vi "2D-ShapeBuilder-INO.vi"(11 "Number of Sides":i32=3) -> (2 "Y out":dbl[](array[numeric])=[1.0, -0.4999999999999998, -0.5000000000000004, 1.0], 3 "X out":dbl[](array[numeric])=[0.0, 0.8660254037844387, -0.8660254037844384, 0.0])   [LabVIEW 2014]
doc: "André Romero - 2018\nandretec@ifsc.usp.br\n\n2D Shape Builder"
panel:
  out "Frequency (KHz)":ext
  out "interval time (us)":ext
  out "Delta Y":dbl[](array[numeric])=[-2999.9999999999995, -1.3642420526593924e-12, 3000.000000000001]
  out "Delta X":dbl[](array[numeric])=[1732.0508075688774, -3464.1016151377544, 1732.0508075688767]
  out "array w/ subset deleted 2":dbl[](array[numeric])=[-999.9999999999995, -1000.0000000000009, 2000.0]
  out "array w/ subset deleted":ext[](array[numeric])=[1732.0508075688774, -1732.0508075688767, 0.0]
  out "Vy":ext[](array[numeric])=[0.04330127018922192983, 1.9691137908567695728e-17, 0.04330127018922193538]
  out "Vx":ext[](array[numeric])=[0.025000000000000005552, 0.05, 0.024999999999999986123]
  in  "Velocidade (mm/s)":ext=0.05
  in  "Radius (steps)":dbl=2000.0
  out "XY Graph 2":cluster{dbl[], dbl[]}(graph)={[0.0, 1732.0508075688774, -1732.0508075688767, 0.0], [2000.0, -999.9999999999995, -1000.0000000000009, 2000.0]}
  out "Y":dbl[](array[numeric])=[2000.0, -999.9999999999995, -1000.0000000000009, 2000.0]
  out "X":dbl[](array[numeric])=[0.0, 1732.0508075688774, -1732.0508075688767, 0.0]
  out "XY Graph":cluster{dbl[], dbl[]}(graph)={[0.0, 0.8660254037844387, -0.8660254037844384, 0.0], [1.0, -0.4999999999999998, -0.5000000000000004, 1.0]}
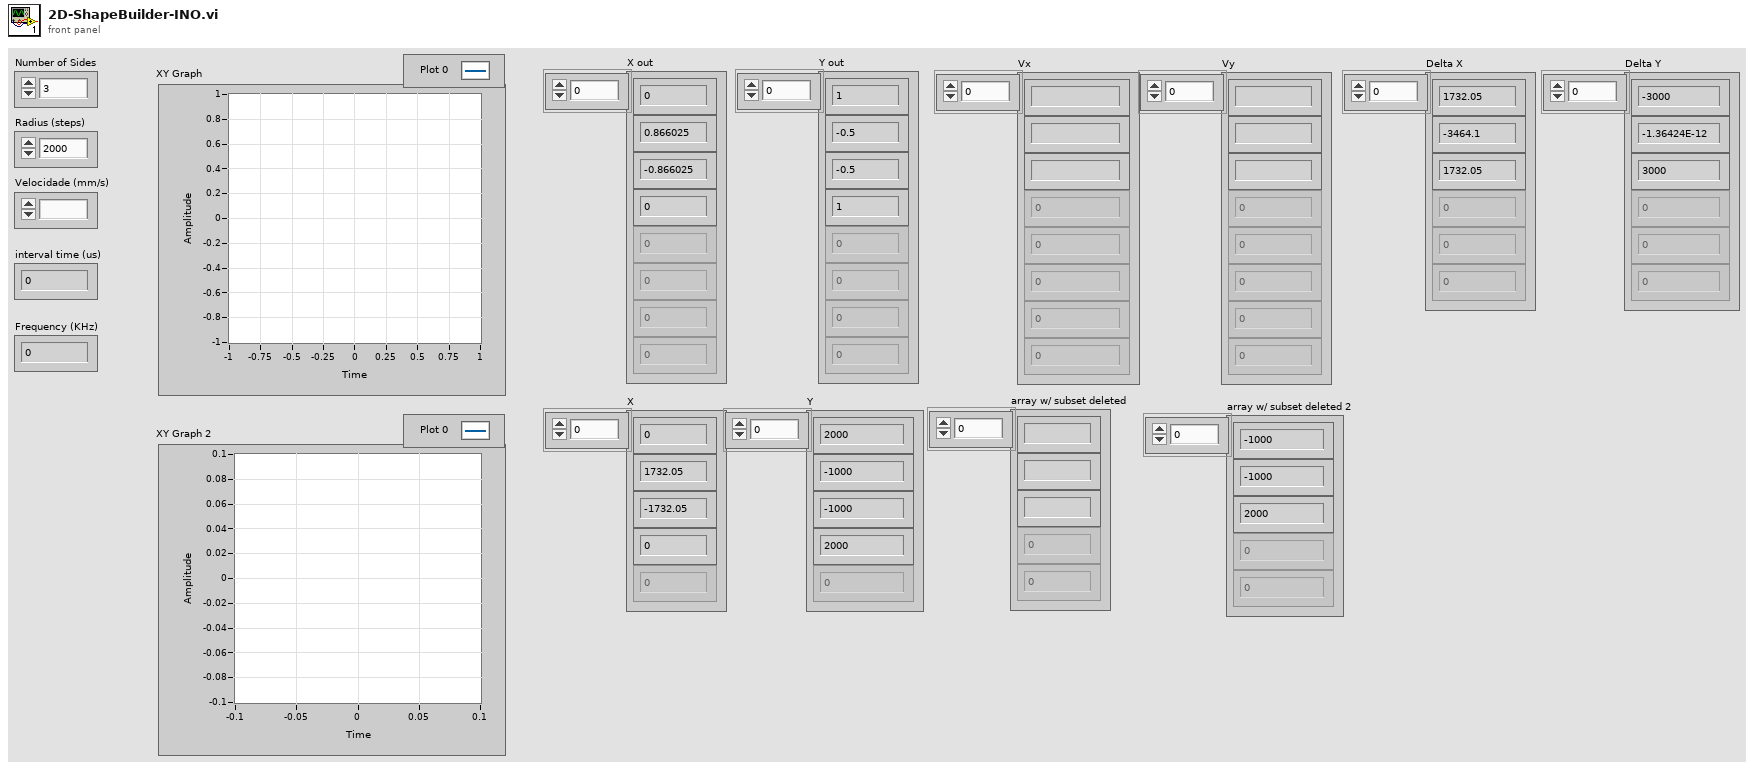
[diagram p1: front panel]
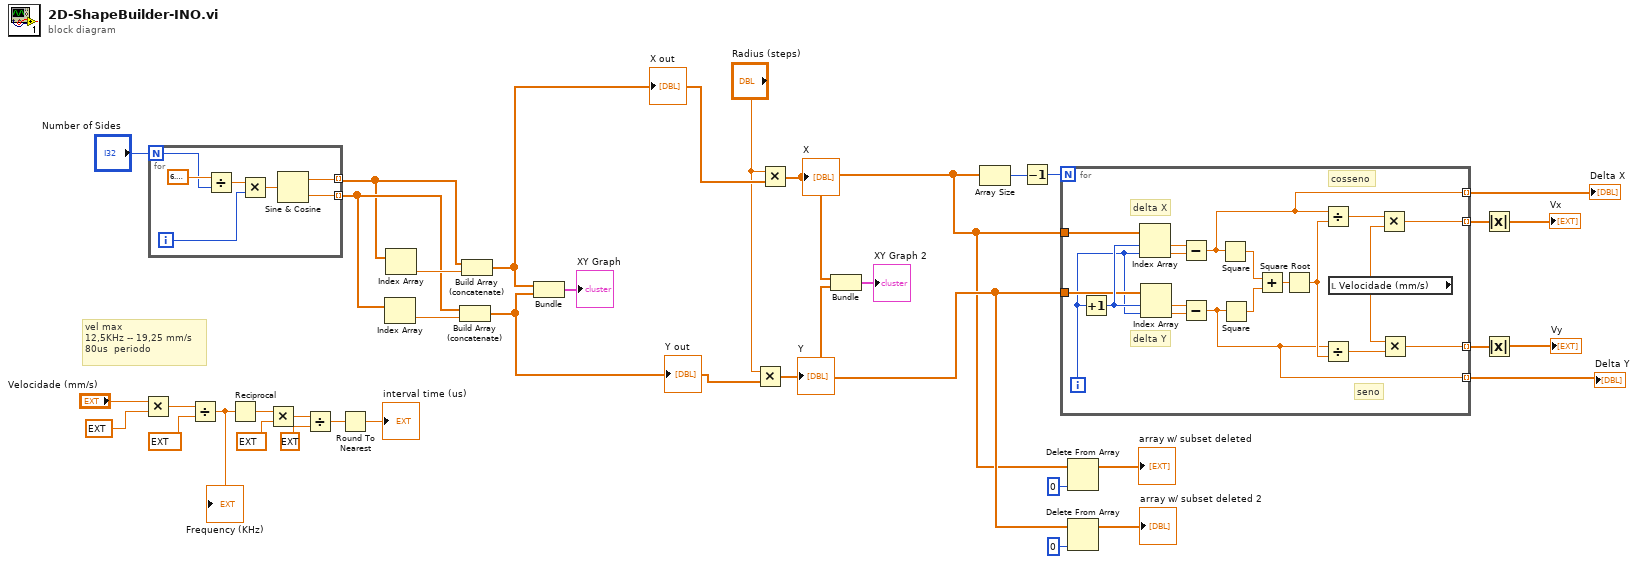
[diagram p0: block diagram]
diagram:
  # "vel max\n12,5KHz -- 19,25 mm/s\n80us  periodo"
  n1 = Multiply(x="Velocidade (mm/s)", y=ext 12.5) -> (x*y=w14:ext)
  n2 = for {
    N: "Number of Sides" -> [w41]
    tunnel: [w37] -> w30 mode=indexing
    tunnel: [w36] -> w31 mode=indexing
    i -> [w39]
    n3 = Divide(x=6.283185307179586, y=w41) -> (x/y=w40:dbl)
    n4 = Multiply(x=w40, y=w39) -> (x*y=w38:dbl)
    n5 = Sine & Cosine(0:w38) -> (1:w37:dbl, 2:w36:dbl)
  }
  n6 = Divide(x=w14, y=ext 19.25) -> (x/y=w12:ext)
  "Frequency (KHz)" <- w12
  n7 = Reciprocal(x=w12) -> (1/x=w11:ext)
  n8 = Multiply(x=w11, y=ext 1000.0) -> (x*y=w9:ext)
  n9 = Divide(x=w9, y=ext 2.0) -> (x/y=w7:ext)
  n10 = Round To Nearest(number=w7) -> (nearest integer value=→"interval time (us)":ext)
  n11 = Index Array(array=w31) -> (element=w32:dbl)  [unwired: 1 in]
  n12 = Index Array(array=w30) -> (element=w33:dbl)  [unwired: 1 in]
  n13 = Build Array (concatenate)(w31, w32) -> (w28:dbl[])
  "Y out" <- w28
  n14 = Build Array (concatenate)(w30, w33) -> (w29:dbl[])
  "X out" <- w29
  n15 = Bundle(w29, w28) -> (→"XY Graph":cluster{dbl[], dbl[]})  [unwired: 1 in]
  n16 = Multiply(x="Radius (steps)", y=w28) -> (x*y=w17:dbl[])
  "Y" <- w17
  n17 = Multiply(x="Radius (steps)", y=w29) -> (x*y=w5:dbl[])
  "X" <- w5
  n18 = Bundle(w5, w17) -> (→"XY Graph 2":cluster{dbl[], dbl[]})  [unwired: 1 in]
  n19 = Array Size(array=w5) -> (size(s)=w25:i32)
  n20 = Decrement(x=w25) -> (x-1=w22:i32)
  n21 = for {
    N: w22 -> [_]
    tunnel: w5 -> [w50]
    tunnel: w17 -> [w49]
    tunnel: [w47] -> w24 mode=indexing
    tunnel: [w46] -> w23 mode=indexing
    tunnel: [w45] -> w4 mode=indexing
    tunnel: [w44] -> w3 mode=indexing
    i -> [w48]
    # "seno"
    # "cosseno"
    # "delta Y"
    # "delta X"
    n22 = Increment(x=w48) -> (x+1=w61:i32)
    n23 = Index Array(array=w50, index #1=w61, index #2=w48) -> (element #1=w52:dbl, element #2=w59:dbl)
    n24 = Index Array(array=w49, index #1=w61, index #2=w48) -> (element #1=w51:dbl, element #2=w60:dbl)
    n25 = Subtract(x=w52, y=w59) -> (x-y=w45:dbl)
    n26 = Subtract(x=w51, y=w60) -> (x-y=w44:dbl)
    n27 = Square(x=w45) -> (x^2=w58:dbl)
    n28 = Square(x=w44) -> (x^2=w57:dbl)
    n29 = Add(x=w58, y=w57) -> (x+y=w56:dbl)
    n30 = Square Root(x=w56) -> (sqrt(x)=w55:dbl)
    n31 = Divide(x=w45, y=w55) -> (x/y=w54:dbl)
    n32 = Divide(x=w44, y=w55) -> (x/y=w53:dbl)
    n33 = local read "Velocidade (mm/s)"() -> (w43:ext)
    n34 = Multiply(x=w54, y=w43) -> (x*y=w47:ext)
    n35 = Multiply(x=w43, y=w53) -> (x*y=w46:ext)
  }
  "Delta X" <- w4
  "Delta Y" <- w3
  n36 = Delete From Array(array=w5, index=0) -> (array with subset deleted=→"array w/ subset deleted":dbl[])  [unwired: 1 in, 1 out]
  n37 = Delete From Array(array=w17, index=0) -> (array with subset deleted=→"array w/ subset deleted 2":dbl[])  [unwired: 1 in, 1 out]
  n38 = Absolute Value(x=w24) -> (abs(x)=→"Vx":ext[])
  n39 = Absolute Value(x=w23) -> (abs(x)=→"Vy":ext[])
